vi "HP1200_get_rotation_speed_set.vi"(7 "device_addr":u16=22, 8 "error in":errorcluster, 11 "conn_id_in":refnum<k5>) -> (0 "error out":errorcluster, 1 "response":string, 2 "rot_speed":i16, 3 "conn_id_out":refnum<k5>, 4 "status":bool)   [LabVIEW 2019]
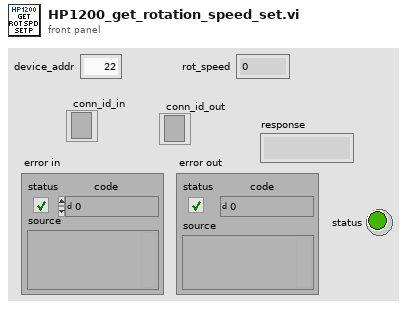
[diagram p1: front panel]
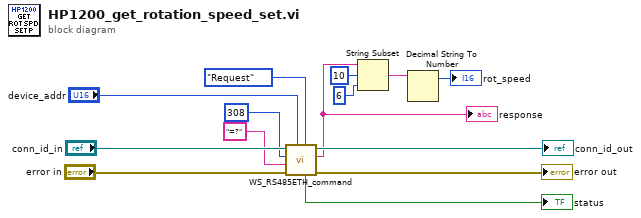
[diagram p0: block diagram]
diagram:
  n1 = call "WS_RS485ETH_command.vi"("action"=enum16{"Request", "Control"}."Request", "device_addr"="device_addr", "error in"="error in", "data_string"="=?" ("data"), "param_num"=u16 308, "conn_id_in"="conn_id_in") -> ("error out"=→"error out":errorcluster, "response"=w5:string, "conn_id_out"=→"conn_id_out":refnum<k5>, "status"=→"status":bool)  [unwired: 2 in]
  "response" <- w5
  n2 = String Subset(string=w5, offset (0)=10, length (rest)=6 ("length (rest)")) -> (substring=w2:string)
  n3 = Decimal String To Number(string=w2) -> (offset past number=→"rot_speed":i32)  [unwired: 2 in, 1 out]
